vi "set_xy.vi"(8 "error in":errorcluster, 10 "y_value_um":dbl format="%0.2f", 11 "x_value_um":dbl format="%0.2f") -> (0 "error out":errorcluster)   [LabVIEW 2018]
uses:
  <vilib>/DAQmx/write.llb/DAQmx Write (Analog 1D DBL NChan 1Samp).vi
  GLOBAL_VAR.vi
  <vilib>/DAQmx/create/channels.llb/DAQmx Create Channel (AO-Voltage-Basic).vi
  <vilib>/DAQmx/miscellaneous.llb/DAQmx Fill In Error Info.vi
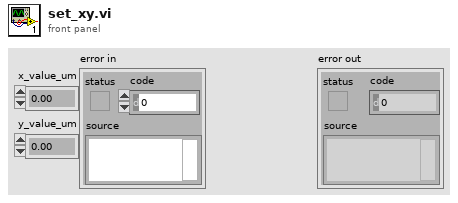
[diagram p1: front panel]
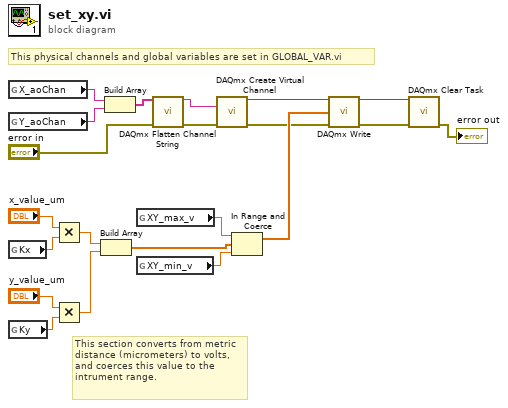
[diagram p0: block diagram]
diagram:
  # "This section converts from metric distance (micrometers) to volts, and coerces this value to the intrument range."
  # "This physical channels and global variables are set in GLOBAL_VAR.vi"
  n1 = global read "GLOBAL_VAR.vi" "X_aoChan"() -> (w19:tag)
  n2 = global read "GLOBAL_VAR.vi" "Y_aoChan"() -> (w20:tag)
  n3 = global read "GLOBAL_VAR.vi" "Kx"() -> (w3:dbl)
  n4 = global read "GLOBAL_VAR.vi" "Ky"() -> (w2:dbl)
  n5 = Multiply(x="x_value_um", y=w3) -> (x*y=w6:dbl)
  n6 = Multiply(x="y_value_um", y=w2) -> (x*y=w5:dbl)
  n7 = Build Array(w6, w5) -> (w7:dbl[])
  n8 = Build Array(w19, w20) -> (w16:tag[])
  n9 = global read "GLOBAL_VAR.vi" "XY_max_v"() -> (w9:dbl)
  n10 = global read "GLOBAL_VAR.vi" "XY_min_v"() -> (w8:dbl)
  n11 = call <vilib>:"DAQmx Flatten Channel String.vi"("names in"=w16, "error in"="error in") -> ("names out"=w15:string, "error out"=w13:errorcluster)  [unwired: 12 in]
  n12 = call-poly <vilib>:"DAQmx Create Virtual Channel.vi"("physical channels"=w15, "error in"=w13) -> ("task out"=w17:refnum<k21>, "error out"=w12:errorcluster)  [unwired: 12 in]
  n13 = In Range and Coerce(upper limit=w9, x=w7, lower limit=w8) -> (coerced(x)=w21:dbl[])  [unwired: 1 out]
  n14 = call-poly <vilib>:"DAQmx Write.vi"("task/channels in"=w17, "data"=w21, "error in"=w12) -> ("task out"=w18:refnum<k21>, "error out"=w11:errorcluster)  [unwired: 10 in, 1 out]
  n15 = call <vilib>:"DAQmx Clear Task.vi"("task in"=w18, "error in"=w11) -> ("error out"=→"error out":errorcluster)  [unwired: 13 in]
